vi "scale to wfm.vi"(0 "reference in":refnum<class "Force Curve_tdms.lvclass">, 2 "Raw data":waveform(dbl)[](array[waveform]), 5 "error in (no error)":errorcluster) -> (14 "reference out":refnum<class "Force Curve_tdms.lvclass">, 16 "wfms out":waveform(dbl)[](array[waveform]), 19 "error out":errorcluster)   [LabVIEW 2019, in "Force Curve_tdms.lvclass"]
uses:
  Force Curve_tdms.lvclass
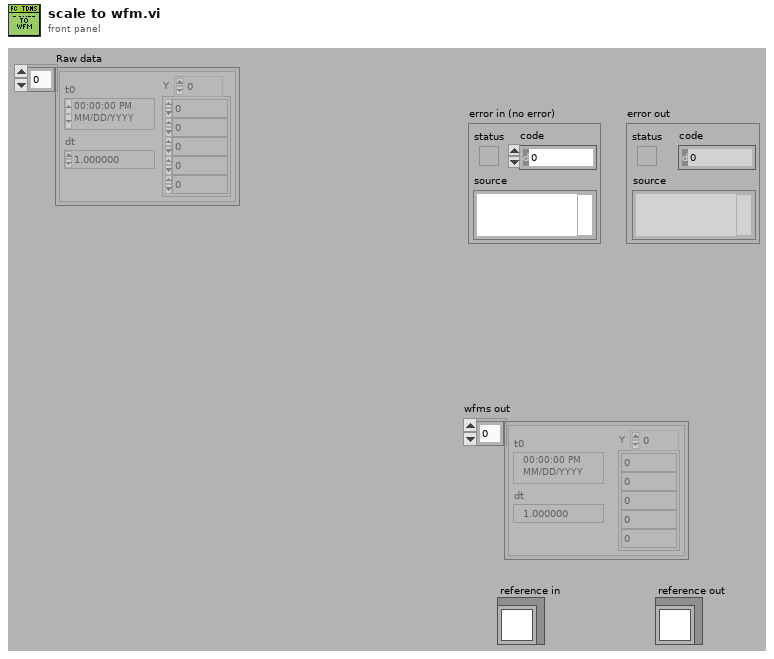
[diagram p1: front panel]
types:
  T1 = typedef "Force Curve_tdms.lvclass/ObjectAttributesRef.ctl" = refnum<data-value>
  T2 = typedef "Force Curve_tdms.lvclass/ObjectAttributes.ctl" = cluster{"MyAttribute":dbl, "Processed data":waveform(dbl)[], "Fcurve Raw Metadata":T3, "Fcurve Metadata":T4, "Fcurve index":T5, "Tau Delay (ms)":dbl, "Contact Spread of dev":dbl, "Fcurve":T6}
  T3 = typedef "TDMS_DataHandler.lvclass/Fcurve Meta data.ctl" = cluster{"property names":string[], "property values":variant[]}
  T4 = typedef "Force Curve_tdms.lvclass/Fcurve Meta data analysis.ctl" = cluster{"dt (us)":dbl, "Dec Factor":dbl, "Z piezo Sensitivity (nm/V)":dbl, "K (N/m)":dbl, "Sp (V)":dbl, "Contact (ms)":dbl, "Zpos contact":dbl, "Vel_app (nm/s)":dbl, "Vel_ret (nm/s)":dbl, "deltaV (nm)":dbl, "Def_V0 (v)":dbl, "Decimating Factor":dbl}
  T5 = typedef "Force Curve_tdms.lvclass/Fcurve Index .ctl" = cluster{"Setpoint index":i32, "Max force index":i32, "Contact point index":i32, "Appoach indices":cluster{"Start":i32, "End":i32}, "Contact indices":cluster{"Start":i32, "End":i32}, "Retract indices":cluster{"Start":i32, "End":i32}}
  T6 = typedef "Force Curve_tdms.lvclass/Force Curve data.ctl" = cluster{"Approach":cluster{"X":dbl[], "Y":dbl[]}, "Contact":cluster{"X":dbl[], "Y":dbl[]}, "Retract":cluster{"X":dbl[], "Y":dbl[]}}
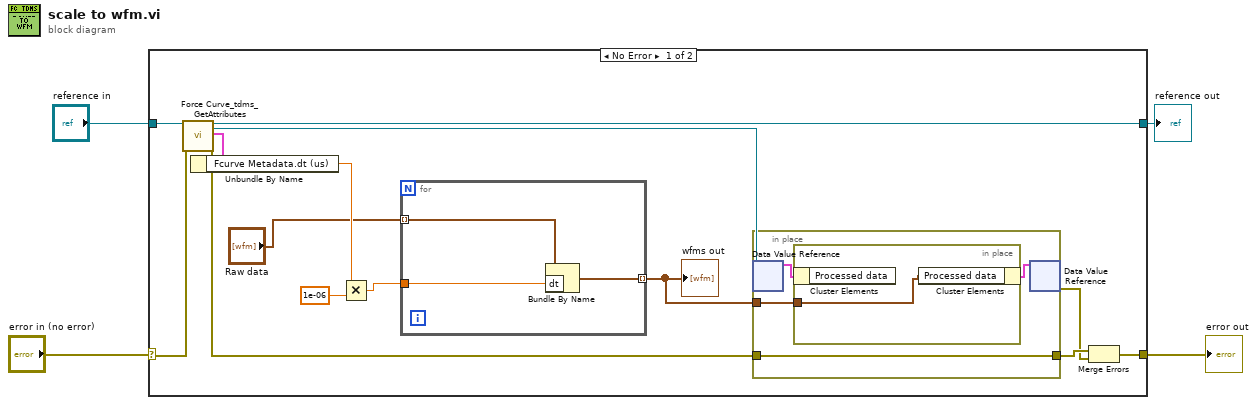
[diagram p0: block diagram]
diagram:
  n1 = case shown="No Error" "error in (no error)" {
    selector: "error in (no error)" -> [w15 w28]
    tunnel: [w18 w28] -> w1
    tunnel: [w16 w27] -> w3
    tunnel: "reference in" -> [w17 w27]
    frame No Error {
      n2 = call "Force Curve_tdms_GetAttributes.vi"("reference in"=w17, "error in (no error)"=w15) -> ("reference out"=w16:refnum<class "Force Curve_tdms.lvclass">, "attributes ref"=w10:T1, "attributes"=w13:T2, "error out"=w14:errorcluster)  [unwired: 14 in]
      n3 = Unbundle By Name(w13) -> ("Fcurve Metadata.dt (us)"=w7:dbl)
      n4 = Multiply(x=w7, y=1e-06) -> (x*y=w9:dbl)
      n5 = for {
        tunnel: "Raw data" -> [w21] mode=indexing
        tunnel: [w20] -> w6 mode=indexing
        tunnel: w9 -> [w19]
        n6 = Bundle By Name(cluster=w21, "dt"=w19) -> (w20:waveform(dbl))
      }
      "wfms out" <- w6
      n7 = in-place {
        in-place-border: w14 -> [w23]
        in-place-border: [w23] -> w12
        in-place-border: w6 -> [w22]
        n8 = in-place-dvr #1(w10) -> (w24:T2)  [unwired: 1 out]
        n9 = in-place {
          in-place-border: w22 -> [w26]
          n10 = in-place-cluster #2(w24) -> ()  [unwired: 1 out]
          n11 = in-place-cluster #2("Processed data"=w26) -> (w25:T2)
        }
        n12 = in-place-dvr #1(w25) -> (w11:errorcluster)  [unwired: 1 out]
      }
      n13 = Merge Errors(w12, w11) -> (w18:errorcluster)
    }
    frame Error {
    }
  }
  "error out" <- w1
  "reference out" <- w3
